vi "Read ROI X-Y.vi"(8 "error in (no error)":errorcluster, 11 "Base Graph in":refnum<class "Base Graph.lvclass">) -> (0 "error out":errorcluster, 2 "ROI XY":T1, 3 "Base Graph out":refnum<class "Base Graph.lvclass">)   [LabVIEW 2023, in "Base Graph.lvclass"]
uses:
  Base Graph.lvclass
  Base Graph.lvclass/Base Graph.ctl
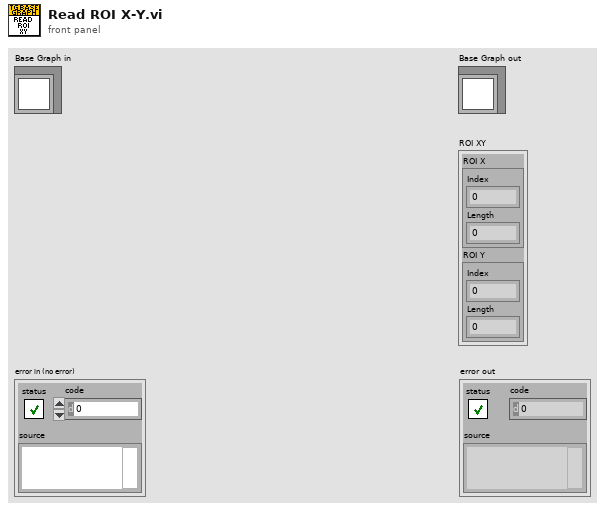
[diagram p1: front panel]
types:
  T1 = cluster{"ROI X":cluster{"Index":u32, "Length":u32}, "ROI Y":cluster{"Index":u32, "Length":u32}}
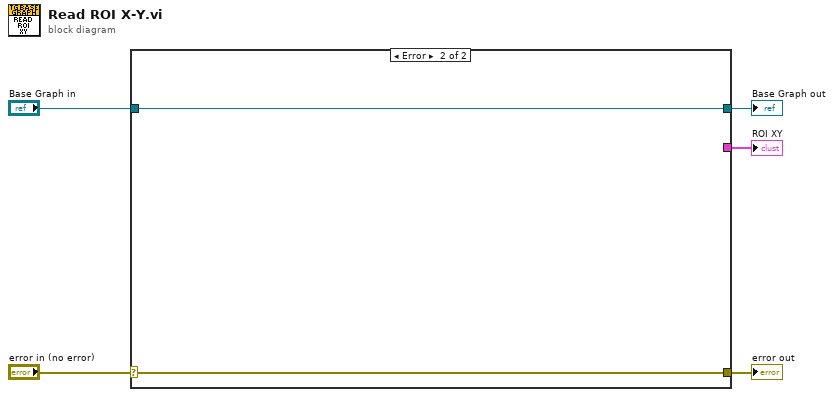
[diagram p0: block diagram]
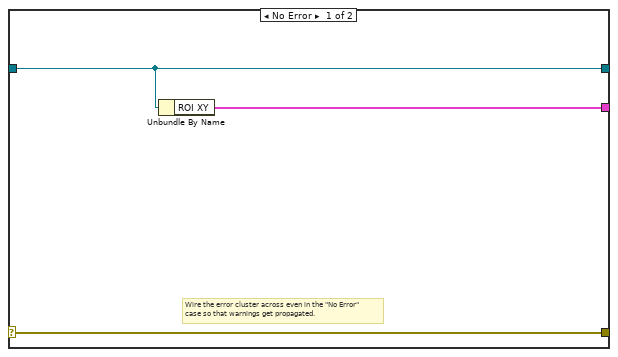
[diagram p2: hidden frame]
diagram:
  n1 = case shown="Error" "error in (no error)" {
    selector: "error in (no error)" -> [w8 w10]
    tunnel: [w8 w10] -> w4
    tunnel: [w7 w9] -> w2
    tunnel: "Base Graph in" -> [w7 w9]
    tunnel: [w6 _] -> w1
    frame No Error {
      # "Wire the error cluster across even in the \"No Error\"\ncase so that warnings get propagated."
      n2 = Unbundle By Name(w7) -> ("ROI XY"=w6:T1)
    }
    frame Error {
    }
  }
  "error out" <- w4
  "Base Graph out" <- w2
  "ROI XY" <- w1
